vi "Calc Scale Specs_modded.vi"(1 "desired font(Application)":T5(ring)=enum."Application Font", 2 "scale definition":T2={"coordinate 1"=5, "value 1"=5.0, "coordinate 2"=5, "value 2"=5.0, "log?(F)"=FALSE, "fmt and prec"={"format"=enum."Hex", "precision"=0}} {"value 2" format="%0.2f"; "value 1" format="%0.2f"}, 3 "scale attributes":T3={"horizontal"=TRUE, "left/top"=FALSE, "draw bar"=FALSE, "line color"=0, "text color(black)"=0}, 5 "[user-specified font]":T4) -> (7 "scale specs":cluster{"coordinate":i16, "label":string}[](array[cluster])=[{"coordinate"=7, "label"="1"}, {"coordinate"=23, "label"="2"}])   [LabVIEW 2018]
doc: "Takes a specification for a Cartesian style scale and calculates the coordinates and labels to use for the scale."
uses:
  fmt_prec_modded.ctl
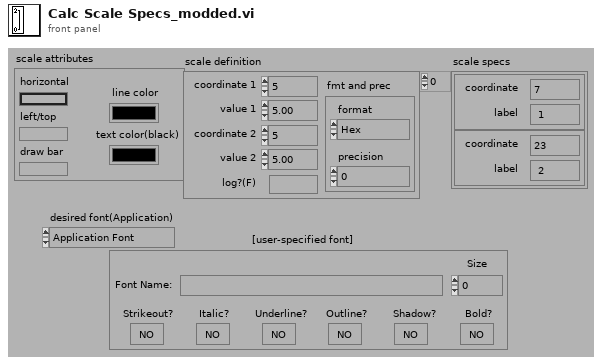
[diagram p1: front panel]
types:
  T1 = typedef "fmt_prec_modded.ctl" = cluster{"format":enum8{"Decimal", "Scientific", "Engineering", "Binary", "Octal", "Hex", "Timestamp"}, "precision":u8}
  T2 = cluster{"coordinate 1":i16, "value 1":dbl, "coordinate 2":i16, "value 2":dbl, "log?(F)":bool, "fmt and prec":T1}
  T3 = cluster{"horizontal":bool, "left/top":bool, "draw bar":bool, "line color":u32, "text color(black)":u32}
  T4 = cluster{"Font Name:":string, "Size":i16, "Strikeout?":bool, "Italic?":bool, "Underline?":bool, "Outline?":bool, "Shadow?":bool, "Bold?":bool}
  T5 = enum16{"User-specified Font", "Application Font", "System Font", "Dialog Font"}
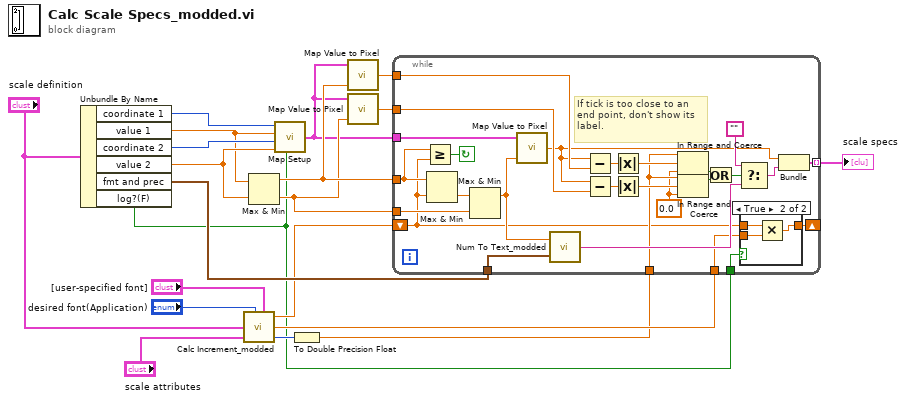
[diagram p0: block diagram]
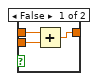
[diagram p2: hidden frame]
diagram:
  n1 = Unbundle By Name("scale definition") -> ("coordinate 1"=w11:i16, "value 1"=w12:dbl, "coordinate 2"=w16:i16, "value 2"=w17:dbl, "fmt and prec"=w18:T1, "log?(F)"=w2:bool)
  n2 = call "Calc Increment_modded.vi"("desired font(Application)"="desired font(Application)", "scale definition"="scale definition", "scale attributes"="scale attributes", "[user-specified font]"="[user-specified font]") -> ("start"=w4:dbl, "increment"=w19:dbl, "text size"=w15:i16)  [unwired: 3 in]
  n3 = Max & Min(x=w12, y=w17) -> (max(x,y)=w14:dbl, min(x,y)=w13:dbl)
  n4 = call <vilib>:"Map Setup.vi"("coordinate 1"=w11, "value 1"=w12, "coordinate 2"=w16, "value 2"=w17, "log?(F)"=w2) -> ("scale factors"=w10:cluster{"a":dbl, "b":dbl, "log?(F)":bool})
  n5 = To Double Precision Float(number=w15) -> (double precision float=w1:dbl)
  n6 = call <vilib>:"Map Value to Pixel.vi"("x"=w14, "scale factors"=w10) -> ("pixel"=w9:dbl)  [unwired: 1 in]
  n7 = call <vilib>:"Map Value to Pixel.vi"("x"=w13, "scale factors"=w10) -> ("pixel"=w8:dbl)  [unwired: 1 in]
  n8 = while {
    tunnel: w2 -> [w21]
    tunnel: w8 -> [w31]
    tunnel: w9 -> [w39]
    tunnel: w1 -> [w30]
    tunnel: w18 -> [w42]
    tunnel: [w46] -> w3 mode=indexing
    tunnel: w19 -> [w24]
    tunnel: w10 -> [w41]
    tunnel: w13 -> [w44]
    tunnel: w14 -> [w43]
    shift-left: w4 -> [w23]
    shift-right: [w22] -> _
    stop <- w45 continue-if-true
    w29 = 0.0
    # "If tick is too close to an\nend point, don't show its\nlabel."
    n9 = Greater Or Equal?(x=w43, y=w23) -> (x >= y?=w45:bool)
    n10 = Max & Min(x=w43, y=w23) -> (min(x,y)=w47:dbl)  [unwired: 1 out]
    n11 = Max & Min(x=w47, y=w44) -> (max(x,y)=w40:dbl)  [unwired: 1 out]
    n12 = call <vilib>:"Map Value to Pixel.vi"("x"=w40, "scale factors"=w41) -> ("pixel"=w25:dbl)  [unwired: 1 in]
    n13 = call "Num To Text_modded.vi"("fmt and prec"=w42, "number"=w40) -> ("numeric string"=w35:string)
    n14 = Subtract(x=w25, y=w39) -> (x-y=w38:dbl)
    n15 = Subtract(x=w25, y=w31) -> (x-y=w32:dbl)
    n16 = Absolute Value(x=w38) -> (abs(x)=w37:dbl)
    n17 = Absolute Value(x=w32) -> (abs(x)=w33:dbl)
    n18 = In Range and Coerce(upper limit=w30, x=w37, lower limit=w29) -> (In Range?=w27:bool)  [unwired: 1 out]
    n19 = In Range and Coerce(upper limit=w30, x=w33, lower limit=w29) -> (In Range?=w26:bool)  [unwired: 1 out]
    n20 = Or(x=w27, y=w26) -> (x .or. y?=w28:bool)
    n21 = Select(t="", s=w28, f=w35) -> (s? t:f=w34:string)
    n22 = case shown="True" w21 {
      tunnel: w24 -> [w49 w53]
      tunnel: w23 -> [w48 w52]
      tunnel: [w50 w51] -> w22
      frame False {
        n23 = Add(x=w48, y=w49) -> (x+y=w50:dbl)
      }
      frame True {
        n24 = Multiply(x=w52, y=w53) -> (x*y=w51:dbl)
      }
    }
    n25 = Bundle("pixel"=w25, "numeric string"=w34) -> (w46:cluster{"pixel":dbl, "numeric string":string})  [unwired: 1 in]
  }
  "scale specs" <- w3
